vi "Acquisition Example.vi"() -> ()   [LabVIEW 2025, in "GettingStarted_Acq_148X_Host.lvlib"]
uses:
  GettingStarted_Acq_148X_Host.lvlib
  Common/Types/Packet Table.ctl
  <instrlib>/FlexRIO/CSI-2/v2/Common/Types/LLP Data Type.ctl
  <vilib>/userDefined/Silver/nirio_resource_slv.ctl
  Types/CSI-2 Data Source.ctl
  Common/Types/Serial Channel Configuration.ctl
  <instrlib>/FlexRIO/CSI-2/v2/FPGA/Types/Display Parameters.ctl
  Common/Types/RAW Interpretation for Display.ctl
  <instrlib>/FlexRIO/CSI-2/v2/FPGA/Types/Timestamp ID.ctl
  Common/Types/GPIO Filter.ctl
  FPGA/Common/Types/SerDes Identifier.ctl
  <instrlib>/FlexRIO/CSI-2/v2/FPGA/Types/GPIO Bank.ctl
  <vilib>/vision/Image Controls.llb/IMAQ Image.ctl
  <vilib>/Utility/miscctls.llb/LVRowAndColumnUnsignedTypeDef.ctl
  <instrlib>/FlexRIO/API/Host/v1/NI FlexRIO/API/Wait for PoC Safe to Disconnect Channels Array.vi
  <vilib>/FPGAPlugInAG/Dynamic/niLvFpga_Close_Dynamic.vi
  <vilib>/rvi/interface/nirviCloseFPGA/nirviCloseFPGA.xnode
  <instrlib>/FlexRIO/API/Host/v1/NI FlexRIO API v1.lvlib
  Common/GettingStarted_Common_148X_Host.lvlib
  <instrlib>/FlexRIO/CSI-2/v2/Common/NI CSI-2 API Common v2.lvlib
  <instrlib>/FlexRIO/CSI-2/v2/FPGA/NI CSI-2 API FPGA v2.lvlib
  FPGA/Common/GettingStarted_Common_148X_FPGA.lvlib
panel:
  in  "Array":u8[](array[numeric])
  out "Acquisition Stopped":bool
  in  "Configuration":T1(tab)
  in  "Logged Packets to Display":i64=1400
  in  "Log Packets to Disk":bool
  in  "Bitfile Path":path=path "C:/dev/hardware-validation/src/labview/auto-vision/Automotive Vision/1487 HIHO GSE/FPGA Bitfiles/PXIe_1487_4_In_4_Out_Acq_Tap.lvbitx"
  in  "TDMS File Directory":path
  in  "RIO Device":T2="PXI1Slot2"
  in  "Display Acquired Images":bool=TRUE
  in  "Log I2C to Disk":bool
  in  "Log GPIO to Disk":bool
  in  "Channel Configurations":T3[](array[typedef])=[{"Serial Channel"="SI1", "FPGA Display Parameters"={"virtual channel"=0.0, "payload data type"=enum."RAW 8", "frame skip count"=0, "line skip count"=0, "pixel skip count"=0.0}, "RAW Display Parameters"={"Interpretation"=enum."Grayscale", "Bayer Parameters"={"Pattern"=3, "Algorithm"=0, "Red Gain"=1.0, "Green Gain"=1.0, "Blue Gain"=1.0}}}] {"RAW Display Parameters"."Bayer Parameters"."Blue Gain" min=0.0 max=3.99 step=0.1 format="%_4g"; "RAW Display Parameters"."Bayer Parameters"."Green Gain" min=0.0 max=3.99 step=0.1 format="%_4g"; "RAW Display Parameters"."Bayer Parameters"."Red Gain" min=0.0 max=3.99 step=0.1 format="%_4g"; "RAW Display Parameters"."Bayer Parameters"."Algorithm" items=["Bilinear", "VNG"]; "RAW Display Parameters"."Bayer Parameters"."Pattern" items=["GB", "GR", "BG", "RG"]}
  in  "CSI-2 Data Source":T7=1 items=["Raw", "Corrected"]
  in  "Configuration Script":path=path "C:/dev/hardware-validation/src/labview/auto-vision/Automotive Vision/1487 HIHO GSE/scripts/Image Receiver Scripts/9296A_RAW8.cpp"
  in  "Acquisition Duration (s)":dbl=1.0 format="%#_13g"
  in  "Continuous Acquisition":bool=TRUE
  in  "Data Type Filter":T5[](array[typedef])
  in  "Virtual Channel Filter":fxp<+,4,4>[](array[numeric])
  in  "Invert Data Type Filter":bool
  in  "Invert Virtual Channel Filter":bool
  in  "Enable First and Last Packet Select":bool=TRUE
  in  "Stop Timeout (s)":dbl=1.0
  in  "First Packet Data Type Select":T5
  in  "Last Packet Data Type Select":T5=enum."Frame End"
  in  "Serial Input Active Lane Count":i32(ring)=4 items=["1 Lane"=1, "2 Lanes"=2, "4 Lanes"=4]
  in  "Reference Clock Frequency (Hz)":dbl=25000000.0 format="%#_6p"
  in  "Power Over Coax Source":i32(ring) items=["None", "Internal", "Auxiliary"]
  in  "timestamp filter":T8[](array[typedef])
  in  "GPIO to Display":T9[](array[typedef])
  in  "GPIO Bank Select":T10
  in  "Write GPIO":bool
  in  "GPIO Bank Write":T11
  out "GPIO Bank Read":T11
  out "Acquisition Duration (s)":dbl format="%.1f"
  out "Acquisition In Progress":bool
  out "Power Over Coax Voltage (V)":dbl[](array[numeric]) format="%#.2pV"
  out "Power Over Coax Current (A)":dbl[](array[numeric]) format="%#.2pA"
  in  "Acquired Serial Input Channel Data":T12(tab)
  out "Source Rate (fps)(1st Display)":dbl
  out "Update Rate (fps)(1st Display)":dbl
  in  "Serial Channel (1st Display)":fxp<+,3,3>
  out "1st channel display":T13(plugin-control)
  out "Source Rate (fps)(2nd Display)":dbl
  out "Update Rate (fps)(2nd Display)":dbl
  out "2nd channel display":T13(plugin-control)
  in  "Serial Channel (2nd Display)":fxp<+,3,3>
  out "Bytes Acquired (1st Channel)":i64 format="%#.6p"
  out "Acquired Packets (1st Channel)":T14
  out "Packets Logged (1st Channel)":i64
  out "Bytes Acquired (2nd Channel)":i64 format="%#.6p"
  out "Acquired Packets (2nd Channel)":T14
  out "Packets Logged (2nd Channel)":i64
  out "I2C Timestamps":T14
  out "GPIO Timestamps Waveform":digitalwaveform[](graph)
  out "Error Parsing GPIO Timestamps":bool
  out "Power Over Coax Source In Range":bool[](array[boolean])
  in  "Stop Acquisition":bool
  out "Error Out":errorcluster
  # "Overview: Configure an acquisition for a CSI-2 sensor and transfer the acquired data and timestamps to disk.  \nInstructions: Visit https://ni.com/r/automotive-camera-module-ref for tutorials and reference material on using this example with the PXIe-148X."
  # "Configuration Settings"
  # "Data Output"
  # "Resource Configuration"
  # "Data Output Configuration"
  # "Channel Configuration"
  # "Acquisition Configuration"
  # "First and Last Packet Select Configuration"
  # "Packet Filter Configuration"
  # "Power Over Coax Configuration"
  # "Clocking Configuration"
  # "I2C Timestamp Configuration"
  # "The timestamp filters listed correspond to the I2C traffic for a specific serial channel:\n\nUser24 = SI0\nUser25 = SI1\nUser26 = SI2\nUser27 = SI3\nUser28 = SI4\nUser29 = SI5\nUser30 = SI6\nUser31 = SI7"
  # "GPIO Configuration"
  # "* For additional packet viewing capability, use GettingStarted_Common_148X_Host.lvlib->TDMS File Viewer.vi"
  # "* For additional packet viewing capability, use GettingStarted_Common_148X_Host.lvlib->TDMS File Viewer.vi"
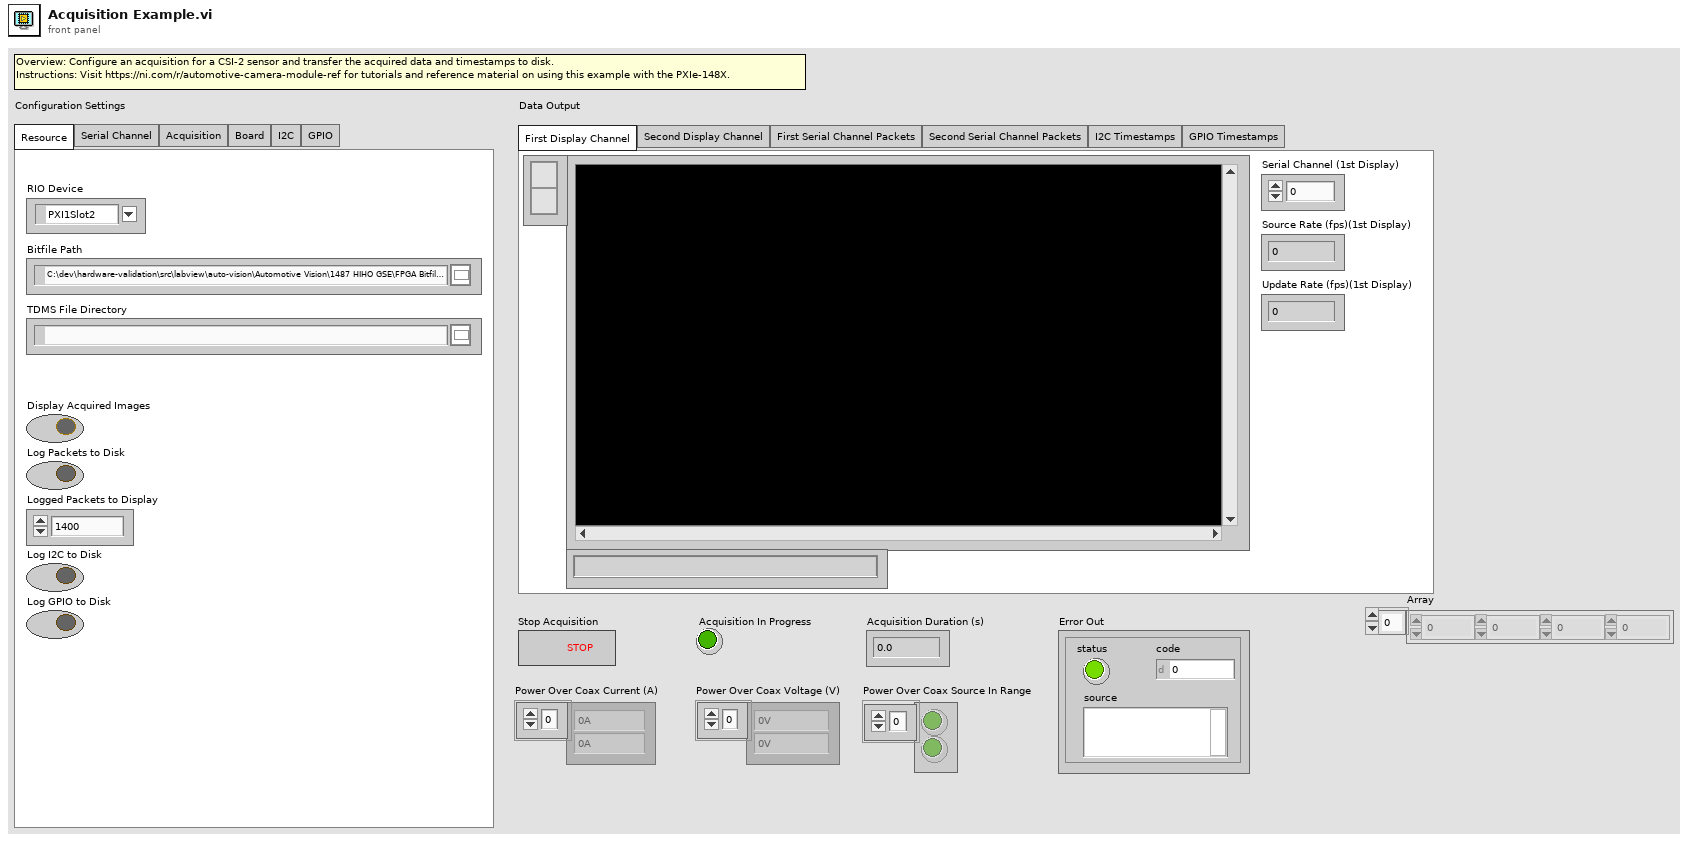
[diagram p1: front panel]
types:
  T1 = enum32{"Resource", "Serial Channel", "Acquisition", "Board", "I2C", "GPIO"}
  T2 = typedef "nirio_resource_slv.ctl" = tag
  T3 = typedef "GettingStarted_Common_148X_Host.lvlib/Serial Channel Configuration.ctl" = cluster{"Serial Channel":string, "FPGA Display Parameters":T4, "RAW Display Parameters":cluster{"Interpretation":T6, "Bayer Parameters":cluster{"Pattern":i32, "Algorithm":i32, "Red Gain":dbl, "Green Gain":dbl, "Blue Gain":dbl}}}
  T4 = typedef "NI CSI-2 API FPGA v2.lvlib/Display Parameters.ctl" = cluster{"virtual channel":fxp<+,4,4>, "payload data type":T5, "frame skip count":u16, "line skip count":u8, "pixel skip count":fxp<+,5,5>}
  T5 = typedef "NI CSI-2 API Common v2.lvlib/LLP Data Type.ctl" = enum8{"Frame Start", "Frame End", "Line Start", "Line End", "End of Transmission", "Reserved 0", "Reserved 1", "Reserved 2", "Generic Short Packet 1", "Generic Short Packet 2", "Generic Short Packet 3", "Generic Short Packet 4", "Generic Short Packet 5", "Generic Short Packet 6", "Generic Short Packet 7", "Generic Short Packet 8", "Null", "Blanking Data", "Embedded 8-bit non Image Data", "Generic Long Packet 1", "Generic Long Packet 2", "Generic Long Packet 3", "Generic Long Packet 4", "Reserved 3", "YUV420 8-bit", "YUV420 10-bit", "Legacy YUV420 8-bit", "Reserved 4", "YUV420 8-bit Chroma Shifted", "YUV420 10-bit Chroma Shifted", "YUV422 8-bit", "YUV422 10-bit", "RGB444", "RGB555", "RGB565", "RGB666", "RGB888", "Reserved 5", "Reserved 6", "RAW 24", "RAW 6", "RAW 7", "RAW 8", "RAW 10", "RAW 12", "RAW 14", "RAW 16", "RAW 20", "User Defined 8-bit Data 1", "User Defined 8-bit Data 2", "User Defined 8-bit Data 3", "User Defined 8-bit Data 4", "User Defined 8-bit Data 5", "User Defined 8-bit Data 6", "User Defined 8-bit Data 7", "User Defined 8-bit Data 8", "USL Command", "Reserved 7", "Reserved 8", "Reserved 9", "Reserved 10", "Reserved 11", "Reserved 12", "LRTE EPD Spacer"}
  T6 = typedef "GettingStarted_Common_148X_Host.lvlib/RAW Interpretation for Display.ctl" = enum16{"Grayscale", "Bayer", "RGB", "YUV422", "YUV420", "Legacy YUV420"}
  T7 = typedef "GettingStarted_Acq_148X_Host.lvlib/CSI-2 Data Source.ctl" = u16
  T8 = typedef "NI CSI-2 API FPGA v2.lvlib/Timestamp ID.ctl" = enum8{"SI0 LLP", "SI1 LLP", "SI2 LLP", "SI3 LLP", "SI4 LLP", "SI5 LLP", "SI6 LLP", "SI7 LLP", "SO0 LLP", "SO1 LLP", "SO2 LLP", "SO3 LLP", "SO4 LLP", "SO5 LLP", "SO6 LLP", "SO7 LLP", "Ser0 GPIO Bank", "Ser1 GPIO Bank", "Ser2 GPIO Bank", "Ser3 GPIO Bank", "Ser4 GPIO Bank", "Ser5 GPIO Bank", "Ser6 GPIO Bank", "Ser7 GPIO Bank", "Des0 GPIO Bank", "Des1 GPIO Bank", "Des2 GPIO Bank", "Des3 GPIO Bank", "Des4 GPIO Bank", "Des5 GPIO Bank", "Des6 GPIO Bank", "Des7 GPIO Bank", "User0", "User1", "User2", "User3", "User4", "User5", "User6", "User7", "User8", "User9", "User10", "User11", "User12", "User13", "User14", "User15", "User16", "User17", "User18", "User19", "User20", "User21", "User22", "User23", "User24", "User25", "User26", "User27", "User28", "User29", "User30", "User31"}
  T9 = typedef "GettingStarted_Common_148X_Host.lvlib/GPIO Filter.ctl" = cluster{"GPIO Bank":T8, "GPIO Number":i32}
  T10 = typedef "GettingStarted_Common_148X_FPGA.lvlib/SerDes Identifier.ctl" = enum8{"None", "SI 0 Deserializer", "SI 1 Deserializer", "SI 2 Deserializer", "SI 3 Deserializer", "SI 4 Deserializer", "SI 5 Deserializer", "SI 6 Deserializer", "SI 7 Deserializer", "SO 0 Serializer", "SO 1 Serializer", "SO 2 Serializer", "SO 3 Serializer", "SO 4 Serializer", "SO 5 Serializer", "SO 6 Serializer", "SO 7 Serializer", "SI 0 SI 1 Deserializer", "SI 2 SI 3 Deserializer", "SI 4 SI 5 Deserializer", "SI 6 SI 7 Deserializer"}
  T11 = typedef "NI CSI-2 API FPGA v2.lvlib/GPIO Bank.ctl" = cluster{"GPIO 0":bool, "GPIO 1":bool, "GPIO 2":bool, "GPIO 3":bool, "GPIO 4":bool, "GPIO 5":bool, "GPIO 6":bool, "GPIO 7":bool, "GPIO 8":bool, "GPIO 9":bool, "GPIO 10":bool}
  T12 = enum32{"First Display Channel", "Second Display Channel", "First Serial Channel Packets", "Second Serial Channel Packets", "I2C Timestamps", "GPIO Timestamps"}
  T13 = typedef "IMAQ Image.ctl" = refnum<image>
  T14 = typedef "GettingStarted_Common_148X_Host.lvlib/Packet Table.ctl" = string[][]
  T15 = typedef "LVRowAndColumnUnsignedTypeDef.ctl" = cluster{"Row":u32, "Column":u32}
  T16 = typedef "GettingStarted_Common_148X_Host.lvlib/Serial Channel Display Parameters.ctl" = cluster{"images":cluster{"grayscale":T13, "color":T13}, "RAW parameters":cluster{"interpretation":T6, "bayer parameters":cluster{"pattern":i32, "algorithm":i32, "red gain":dbl, "green gain":dbl, "blue gain":dbl}}}
  T17 = cluster{"Source Rate (fps)(1st Display)":refnum<vi>, "Update Rate (fps)(1st Display)":refnum<vi>}
  T18 = cluster{"Source Rate (fps)(2nd Display)":refnum<vi>, "Update Rate (fps)(2nd Display)":refnum<vi>}
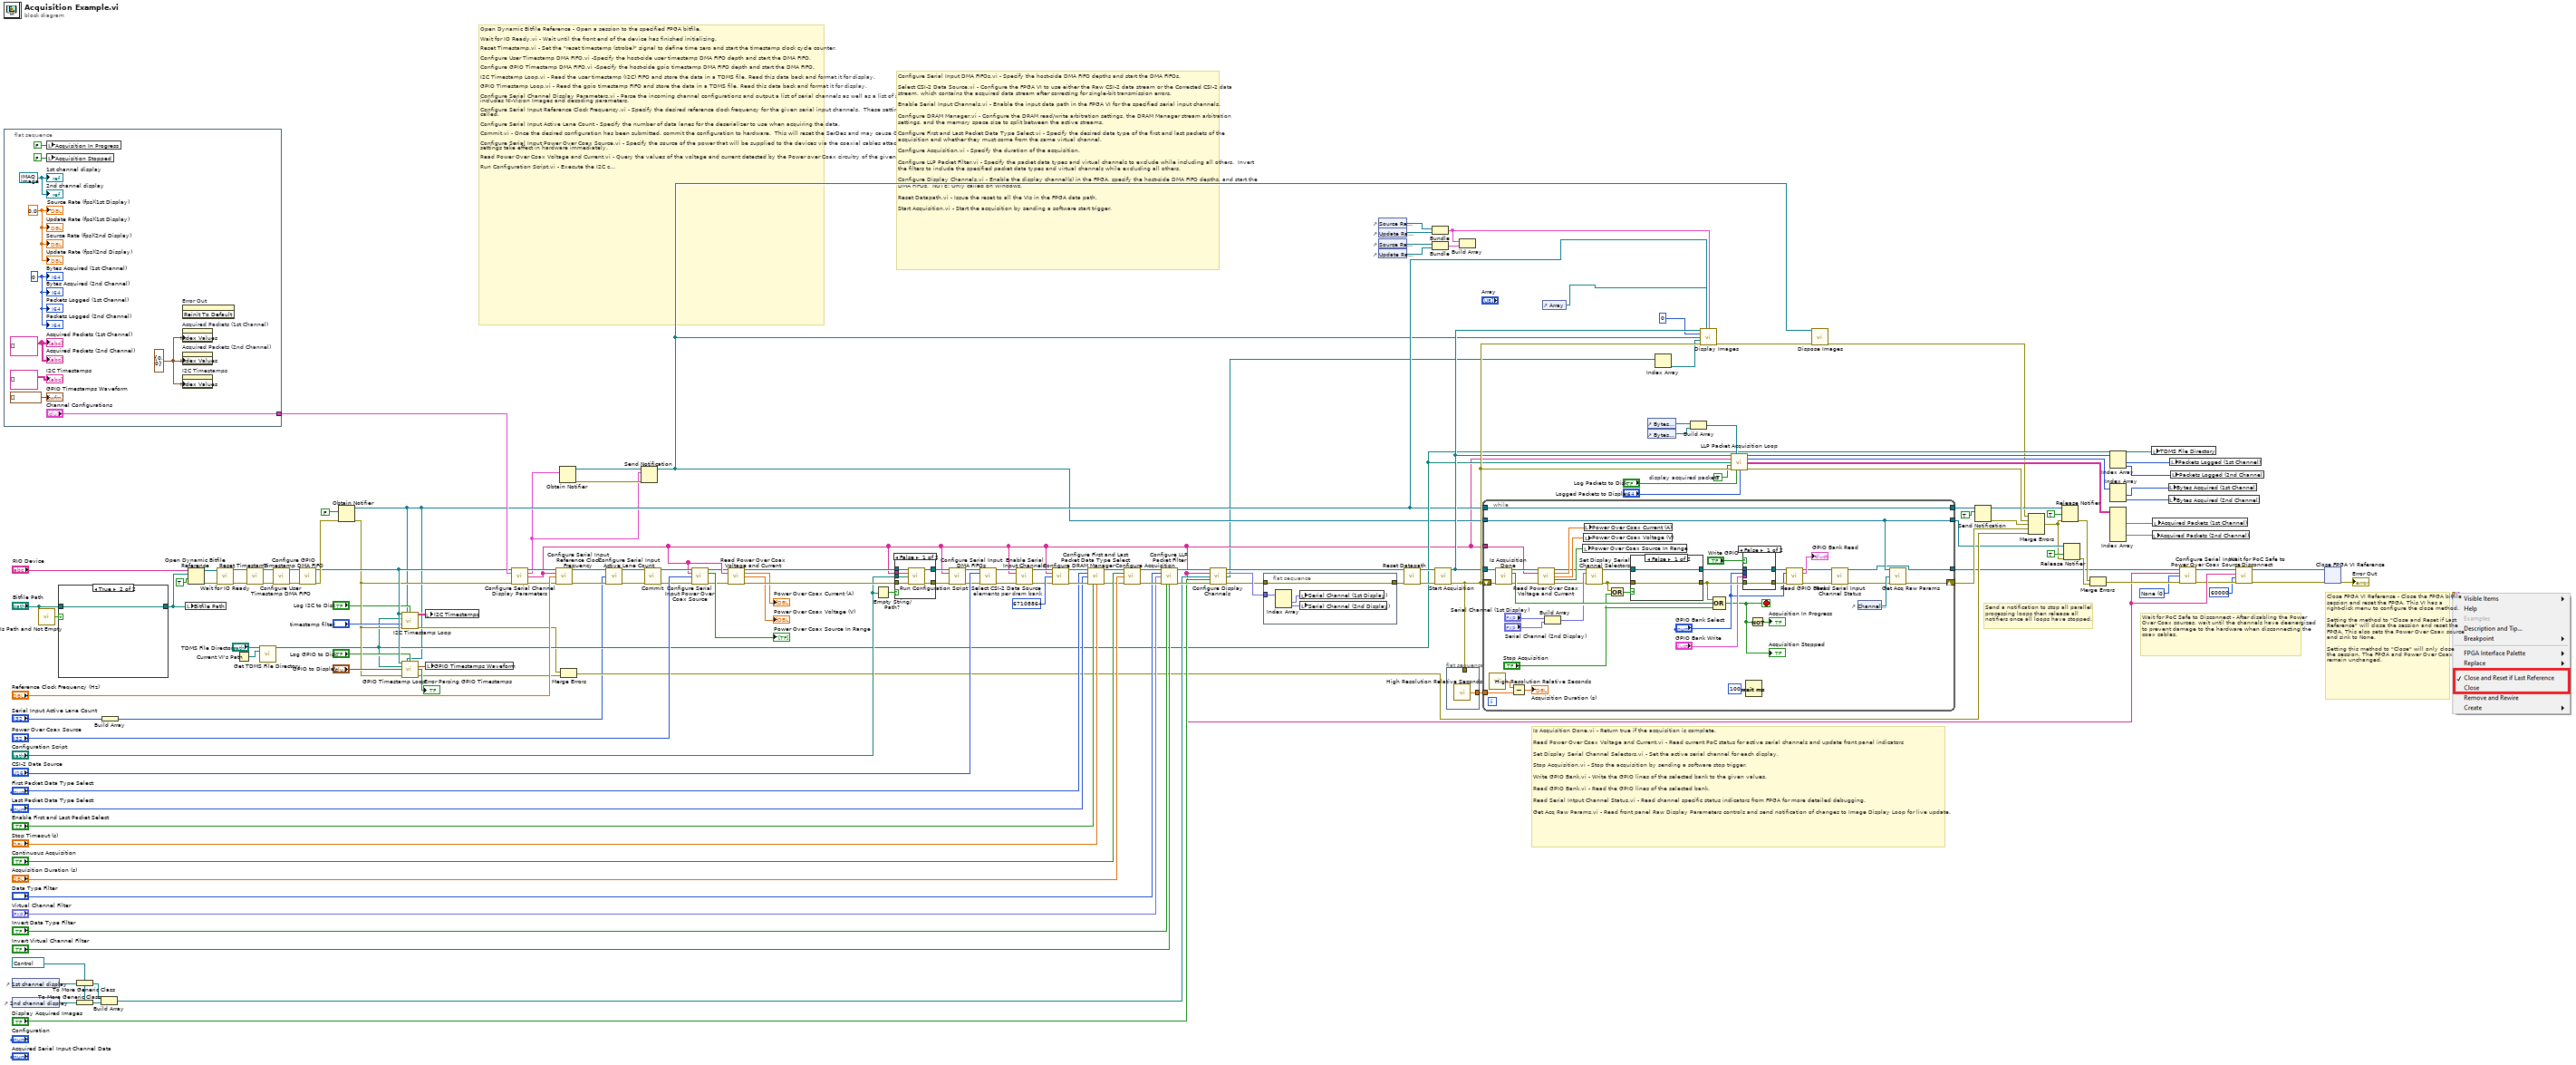
[diagram p0: block diagram]
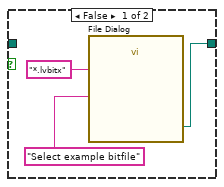
[diagram p2: hidden frame]
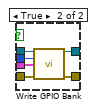
[diagram p4: hidden frame]
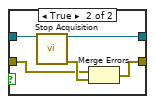
[diagram p5: hidden frame]
diagram:
  w9 = 0 items=["None", "Internal", "Auxiliary"] ("power over coax source")
  w36 = TRUE  # display acquired packets
  w85 = refnum<vi> refnum ("image display reference")
  w150 = u32 67108864  # elements per dram bank
  # "Wait for PoC Safe to Disconnect - After disabling the Power Over Coax sources, wait until the channels have deenergized to prevent damage to the hardware when disconnecting the coax cables."
  # "Send a notification to stop all parallel processing loops then release all notifiers once all loops have stopped."
  # "Configure Serial Input DMA FIFOs.vi - Specify the host-side DMA FIFO depths and start the DMA FIFOs.\n\nSelect CSI-2 Data Source.vi - Configure the FPGA VI to use either the Raw CSI-2 data stream or the Corrected CSI-2 data stream, which contains the acquired data stream after correcting for single-bit transmission errors.\n\nEnable Serial Input Channels.vi - Enable the input data path in the FPGA VI for the specified serial input channels.\n\nConfigure DRAM Manager.vi - Configure the DRAM read/write arbitration settings, the DRAM Manager stream arbitration settings, and the memory space size to split between the active streams.\n\nConfigure First and Last Packet Data Type Select.vi - Specify the desired data type of the first and last packets of the acquisition and whether they must come from the same virtual channel.\n\nConfigure Acquisition.vi - Specify the duration of the acquisition.\n\nConfigure LLP Packet Filter.vi - Specify the packet data types and virtual channels to exclude while including all others.  Invert the filters to include the specified packet data types and virtual channels while excluding all others.\n\nConfigure Display Channels.vi - Enable the display channel(s) in the FPGA, specify the host-side DMA FIFO depths, and start the DMA FIFOs.  NOTE: Only called on Windows. \n\nReset Datapath.vi - Issue the reset to all the VIs in the FPGA data path.\n\nStart Acquisition.vi - Start the acquisition by sending a software start trigger."
  # "Close FPGA VI Reference - Close the FPGA bitfile session and reset the FPGA. This VI has a right-click menu to configure the close method. \n\nSetting the method to \"Close and Reset if Last Reference\" will close the session and reset the FPGA. This also sets the Power Over Coax source and sink to None.\n\nSetting this method to \"Close\" will only close the session. The FPGA and Power Over Coax remain unchanged."
  # "Open Dynamic Bitfile Reference - Open a session to the specified FPGA bitfile.\n\nWait for IO Ready.vi - Wait until the front end of the device has finished initializing.\n\nReset Timestamp.vi - Set the \"reset timestamp (strobe)\" signal to define time zero and start the timestamp clock cycle counter.\n\nConfigure User Timestamp DMA FIFO.vi -Specify the host-side user timestamp DMA FIFO depth and start the DMA FIFO.\n\nConfigure GPIO Timestamp DMA FIFO.vi -Specify the host-side gpio timestamp DMA FIFO depth and start the DMA FIFO.\n\nI2C Timestamp Loop.vi - Read the user timestamp (I2C) FIFO and store the data in a TDMS file. Read this data back and format it for display.\n\nGPIO Timestamp Loop.vi - Read the gpio timestamp FIFO and store the data in a TDMS file. Read this data back and format it for display.\n\nConfigure Serial Channel Display Parameters.vi - Parse the incoming channel configurations and output a list of serial channels as well as a list of serial channel display parameters, which includes NI-Vision Images and decoding parameters.\n\nConfigure Serial Input Reference Clock Frequency.vi - Specify the desired reference clock frequency for the given serial input channels.  These settings do not take effect until Commit.vi is called.\n\nConfigure Serial Input Active Lane Count - Specify the number of data lanes for the deserializer to use when acquiring the data. \n\nCommit.vi - Once the desired configuration has been submitted, commit the configuration to hardware.  This will reset the SerDes and may cause GPIO lines to toggle. \n\nConfigure Serial Input Power Over Coax Source.vi - Specify the source of the power that will be supplied to the devices via the coaxial cables attached to the given serial input channels.  These settings take effect in hardware immediately.\n\nRead Power Over Coax Voltage and Current.vi - Query the values of the voltage and current detected by the Power over Coax circuitry of the given serial channels.\n\nRun Configuration Script.vi - Execute the I2C commands in the specified script file for the given serial channels.  The script is used to configure the serializer, deserializer, or other I2C slave device, such as the image sensor."
  # "Is Acquisition Done.vi - Return true if the acquisition is complete.\n\nRead Power Over Coax Voltage and Current.vi - Read current PoC status for active serial channels and update front panel indicators \n\nSet Display Serial Channel Selectors.vi - Set the active serial channel for each display.\n\nStop Acquisition.vi - Stop the acquisition by sending a software stop trigger.\n\nWrite GPIO Bank.vi - Write the GPIO lines of the selected bank to the given values.\n\nRead GPIO Bank.vi - Read the GPIO lines of the selected bank.\n\nRead Serial Intput Channel Status.vi - Read channel specific status indicators from FPGA for more detailed debugging.\n\nGet Acq Raw Params.vi - Read front panel Raw Display Parameters controls and send notification of changes to Image Display Loop for live update."
  n1 = flat-sequence {
    tunnel: ["Channel Configurations"] -> w98
    frame #0 {
      w151 = T15 {"Row"=0, "Column"=0} ("Index Values")
      w158 = T14 [] ("Acquired Packets (1st Channel)")
      w154 = 0 ("Number of Packets Acquired (1st Channel)")
      w157 = 0.0 ("display fps (2nd display)")
      w160 = T13 refnum ("first channel display")
      n2 = local write "Acquisition In Progress"(FALSE ("Acquisition In Progress")) -> ()
      n3 = local write "Acquisition Stopped"(FALSE ("Acquisition Stopped")) -> ()
      n4 = invoke on="Error Out" class="Clust (strict)" method="Reinit To Default"() -> ()  [unwired: 3 in, 3 out]
      n5 = property on="Acquired Packets (1st Channel)" class="Tbl (strict)"("Index Values"=w151) -> ()  [unwired: 2 in, 2 out]
      n6 = property on="Acquired Packets (2nd Channel)" class="Tbl (strict)"("Index Values"=w151) -> ()  [unwired: 2 in, 2 out]
      n7 = property on="I2C Timestamps" class="Tbl (strict)"("Index Values"=w151) -> ()  [unwired: 2 in, 2 out]
      "1st channel display" <- w160
      "2nd channel display" <- w160
      "Update Rate (fps)(1st Display)" <- w157
      "Update Rate (fps)(2nd Display)" <- w157
      "Acquired Packets (1st Channel)" <- w158
      "Packets Logged (1st Channel)" <- w154
      "Acquired Packets (2nd Channel)" <- w158
      "Packets Logged (2nd Channel)" <- w154
      "Source Rate (fps)(1st Display)" <- w157
      "Source Rate (fps)(2nd Display)" <- w157
      "GPIO Timestamps Waveform" <- digitalwaveform[] [] ("GPIO Timestamps Waveform")
      "I2C Timestamps" <- T14 [] ("I2C Timestamps 2")
      "Bytes Acquired (1st Channel)" <- w154
      "Bytes Acquired (2nd Channel)" <- w154
    }
  }
  n8 = control-ref of="1st channel display"() -> (w95:refnum<vi>)
  n9 = control-ref of="2nd channel display"() -> (w93:refnum<vi>)
  n10 = call <vilib>:"Is Path and Not Empty.vi"("path"="Bitfile Path") -> ("Is Path and Not Empty?"=w132:bool)  [unwired: 4 in]
  n11 = case shown="True" w132 {
    tunnel: "Bitfile Path" -> [_ w164]
    tunnel: [w162 w164] -> w131
    frame False {
      n12 = call "File Dialog"("prompt"="Select example bitfile", "pattern (all files)"="*.lvbitx") -> ("selected path"=w162:path)  [unwired: 10 in, 3 out]
    }
    frame True {
    }
  }
  n13 = To More Generic Class(target class=w85, reference=w95) -> (generic class reference=w94:refnum<vi>)
  n14 = To More Generic Class(target class=w85, reference=w93) -> (generic class reference=w92:refnum<vi>)
  n15 = Build Array(w94, w92) -> (w90:refnum<vi>[])
  n16 = Build Array("Serial Input Active Lane Count") -> (w27:i32[])
  n17 = local write "Bitfile Path"(w131) -> ()
  n18 = Open Dynamic Bitfile Reference(0:"RIO Device", 1:w131, 2:TRUE ("Run When Loaded")) -> (5:w129:refnum<k20>, 8:w130:errorcluster)  [unwired: 2 in]
  n19 = call <instrlib>:"Wait for IO Ready.vi"("fpga interface in"=w129, "error in"=w130) -> ("fpga interface out"=w65:refnum<k20>, "error out"=w66:errorcluster)  [unwired: 10 in, 2 out]
  n20 = Current VI's Path() -> (path=w102:path)
  n21 = call "Reset Timestamp.vi"("fpga interface in"=w65, "error in (no error)"=w66) -> ("fpga interface out"=w55:refnum<k20>, "error out"=w54:errorcluster)  [unwired: 12 in]
  n22 = call "Get TDMS File Directory.vi"("tdms file directory in"="TDMS File Directory", "calling vi path"=w102) -> ("tdms file directory out"=w40:path)  [unwired: 13 in]
  n23 = call "Configure User Timestamp DMA FIFO.vi"("fpga interface in"=w55, "error in (no error)"=w54) -> ("fpga interface out"=w53:refnum<k20>, "error out"=w52:errorcluster)  [unwired: 12 in]
  n24 = call "Configure GPIO Timestamp DMA FIFO.vi"("fpga interface in"=w53, "error in (no error)"=w52) -> ("fpga interface out"=w49:refnum<k20>, "error out"=w51:errorcluster)  [unwired: 12 in]
  n25 = Obtain Notifier(notification data type=FALSE ("result"), error in (no error)=w51) -> (notifier out=w26:refnum<notifier>, error out=w43:errorcluster)  [unwired: 2 in, 1 out]
  n26 = call "I2C Timestamp Loop.vi"("fpga interface in"=w49, "'stop' notifier"=w26, "log i2c to disk"="Log I2C to Disk", "tdms file directory"=w40, "timestamp filter"="timestamp filter", "error in (no error)"=w43) -> ("i2c data"=w48:string[][], "error out"=w38:errorcluster)  [unwired: 8 in]
  n27 = call "GPIO Timestamp Loop.vi"("fpga interface in"=w49, "'stop' notifier"=w26, "log gpio to disk"="Log GPIO to Disk", "tdms file directory"=w40, "gpio to display"="GPIO to Display", "error in (no error)"=w43) -> ("gpio timestamps waveform"=w47:digitalwaveform[], "error parsing gpio timestamps"=→"Error Parsing GPIO Timestamps":bool, "error out"=w37:errorcluster)  [unwired: 7 in]
  n28 = local write "I2C Timestamps"(w48) -> ()
  n29 = local write "GPIO Timestamps Waveform"(w47) -> ()
  n30 = call "Configure Serial Channel Display Parameters.vi"("fpga interface in"=w49, "serial channel configurations"=w98, "error in (no error)"=w43) -> ("fpga interface out"=w97:refnum<k20>, "serial channel display parameters"=w23:T16[], "serial channels"=w12:string[], "error out"=w96:errorcluster)  [unwired: 9 in]
  n31 = call "Configure Serial Input Reference Clock Frequency.vi"("fpga interface in"=w97, "serial input channels"=w12, "serial input reference clock frequency (Hz)"="Reference Clock Frequency (Hz)", "error in (no error)"=w96) -> ("fpga interface out"=w32:refnum<k20>, "error out"=w31:errorcluster)  [unwired: 10 in]
  n32 = Obtain Notifier(notification data type=w23) -> (notifier out=w25:refnum<notifier>, error out=w24:errorcluster)  [unwired: 3 in, 1 out]
  n33 = Merge Errors(w38, w37) -> (w33:errorcluster)
  n34 = call "Configure Serial Input Active Lane Count.vi"("fpga interface in"=w32, "serial input active lane counts"=w27, "error in (no error)"=w31) -> ("fpga interface out"=w30:refnum<k20>, "error out"=w29:errorcluster)  [unwired: 11 in]
  n35 = Send Notification(notification=w23, notifier=w25, error in (no error)=w24) -> (notifier out=w22:refnum<notifier>)  [unwired: 1 out]
  n36 = call <instrlib>:"Commit.vi"("fpga interface in"=w30, "error in"=w29) -> ("fpga interface out"=w136:refnum<k20>, "error out"=w137:errorcluster)  [unwired: 12 in]
  n37 = call "Configure Serial Input Power Over Coax Source.vi"("fpga interface in"=w136, "serial input channels"=w12, "power over coax source"="Power Over Coax Source", "error in (no error)"=w137) -> ("fpga interface out"=w10:refnum<k20>, "power over coax source in range"=→"Power Over Coax Source In Range":bool[], "error out"=w11:errorcluster)  [unwired: 9 in]
  n38 = call "Read Power Over Coax Voltage and Current.vi"("fpga interface in"=w10, "serial channels"=w12, "error in (no error)"=w11) -> ("fpga interface out"=w126:refnum<k20>, "current (A)"=→"Power Over Coax Current (A)":dbl[], "voltage (V)"=→"Power Over Coax Voltage (V)":dbl[], "error out"=w127:errorcluster)  [unwired: 8 in, 1 out]
  n39 = Empty String/Path?(string/path="Configuration Script") -> (empty?=w68:bool)
  n40 = case shown="False" w68 {
    tunnel: [w170 w171] -> w148
    tunnel: [w169 w172] -> w140
    tunnel: w127 -> [w168 w171]
    tunnel: w126 -> [w167 w172]
    tunnel: w12 -> [w166 _]
    tunnel: "Configuration Script" -> [w165 _]
    frame False {
      n41 = call "Run Configuration Script.vi"("fpga interface in"=w167, "serial channels"=w166, "configuration script"=w165, "error in (no error)"=w168) -> ("fpga interface out"=w169:refnum<k20>, "error out"=w170:errorcluster)  [unwired: 10 in]
    }
    frame True {
    }
  }
  n42 = call "Configure Serial Input DMA FIFOs.vi"("fpga interface in"=w140, "serial channels"=w12, "error in (no error)"=w148) -> ("fpga interface out"=w118:refnum<k20>, "error out"=w115:errorcluster)  [unwired: 11 in]
  n43 = call "Select CSI-2 Data Source.vi"("fpga interface in"=w118, "csi-2 data source"="CSI-2 Data Source", "error in (no error)"=w115) -> ("fpga interface out"=w117:refnum<k20>, "error out"=w116:errorcluster)  [unwired: 11 in]
  n44 = call "Enable Serial Input Channels.vi"("fpga interface in"=w117, "serial input channels"=w12, "error in (no error)"=w116) -> ("fpga interface out"=w139:refnum<k20>, "error out"=w149:errorcluster)  [unwired: 11 in]
  n45 = call "Configure DRAM Manager.vi"("fpga interface in"=w139, "serial channels"=w12, "elements per dram bank"=w150, "error in (no error)"=w149) -> ("fpga interface out"=w111:refnum<k20>, "error out"=w114:errorcluster)  [unwired: 10 in]
  n46 = call "Configure First and Last Packet Data Type Select.vi"("fpga interface in"=w111, "first packet data type select"="First Packet Data Type Select", "last packet data type select"="Last Packet Data Type Select", "error in (no error)"=w114, "enable first and last packet select"="Enable First and Last Packet Select", "stop timeout (s)"="Stop Timeout (s)") -> ("fpga interface out"=w112:refnum<k20>, "error out"=w113:errorcluster)  [unwired: 8 in]
  n47 = call "Configure Acquisition.vi"("fpga interface in"=w112, "continuous acquisition (T)"="Continuous Acquisition", "acquisition duration (s)"="Acquisition Duration (s)", "error in (no error)"=w113) -> ("fpga interface out"=w145:refnum<k20>, "error out"=w146:errorcluster)  [unwired: 10 in]
  n48 = call "Configure LLP Packet Filter.vi"("fpga interface in"=w145, "data type filter"="Data Type Filter", "virtual channel filter"="Virtual Channel Filter", "error in (no error)"=w146, "invert data type filter"="Invert Data Type Filter", "invert virtual channel filter"="Invert Virtual Channel Filter") -> ("fpga interface out"=w99:refnum<k20>, "error out"=w91:errorcluster)  [unwired: 8 in]
  n49 = call "Configure Display Channels.vi"("fpga interface in"=w99, "serial channels"=w12, "display references in"=w90, "enable image display"="Display Acquired Images", "error in (no error)"=w91) -> ("fpga interface out"=w89:refnum<k20>, "display serial channels"=w88:fxp<+,3,3>[], "display references out"=w3:refnum<vi>[], "error out"=w87:errorcluster)  [unwired: 7 in]
  n50 = flat-sequence {
    tunnel: w88 -> [w174]
    tunnel: w87 -> [w173]
    tunnel: [w173] -> w86
    frame #0 {
      n51 = Index Array(array=w174) -> (element #1=w176:fxp<+,3,3>, element #2=w175:fxp<+,3,3>)  [unwired: 2 in]
      n52 = local write "Serial Channel (1st Display)"(w176) -> ()
      n53 = local write "Serial Channel (2nd Display)"(w175) -> ()
    }
  }
  n54 = control-ref of="Source Rate (fps)(1st Display)"() -> (w78:refnum<vi>)
  n55 = control-ref of="Update Rate (fps)(1st Display)"() -> (w79:refnum<vi>)
  n56 = control-ref of="Source Rate (fps)(2nd Display)"() -> (w77:refnum<vi>)
  n57 = control-ref of="Update Rate (fps)(2nd Display)"() -> (w76:refnum<vi>)
  n58 = call "Reset Datapath.vi"("fpga interface in"=w89, "error in (no error)"=w86) -> ("fpga interface out"=w147:refnum<k20>, "error out"=w50:errorcluster)  [unwired: 12 in]
  n59 = Bundle("Source Rate (fps)(1st Display)"=w78, "Update Rate (fps)(1st Display)"=w79) -> (w5:T17)  [unwired: 1 in]
  n60 = Bundle("Source Rate (fps)(2nd Display)"=w77, "Update Rate (fps)(2nd Display)"=w76) -> (w75:T18)  [unwired: 1 in]
  n61 = call "Start Acquisition.vi"("fpga interface in"=w147, "error in (no error)"=w50) -> ("fpga interface out"=w63:refnum<k20>, "error out"=w64:errorcluster)  [unwired: 12 in]
  n62 = flat-sequence {
    tunnel: [w177] -> w104
    tunnel: w64 -> [_]
    frame #0 {
      n63 = call <vilib>:"High Resolution Relative Seconds.vi"() -> ("relative seconds"=w177:dbl)
    }
  }
  n64 = Build Array(w5, w75) -> ()  [unwired: 1 out]
  n65 = while {
    shift-right: [w184] -> w34
    shift-left: w64 -> [w186]
    tunnel: w63 -> [w200]
    tunnel: w12 -> [w212]
    tunnel: w104 -> [w207]
    tunnel: w26 -> [w185]
    tunnel: [w185] -> w60
    tunnel: w22 -> [w182]
    tunnel: [w178] -> w16
    tunnel: [w182] -> w20
    stop <- w187 stop-if-true
    n66 = call <vilib>:"High Resolution Relative Seconds.vi"() -> ("relative seconds"=w208:dbl)
    n67 = call "Is Acquisition Done.vi"("fpga interface in"=w200, "error in (no error)"=w186) -> ("fpga interface out"=w213:refnum<k20>, "acquisition done"=w217:bool, "error out"=w214:errorcluster)  [unwired: 11 in]
    n68 = Subtract(x=w208, y=w207) -> (x-y=→"Acquisition Duration (s)":dbl)
    n69 = call "Read Power Over Coax Voltage and Current.vi"("fpga interface in"=w213, "serial channels"=w212, "error in (no error)"=w214) -> ("fpga interface out"=w202:refnum<k20>, "current (A)"=w211:dbl[], "voltage (V)"=w209:dbl[], "in range"=w210:bool[], "error out"=w201:errorcluster)  [unwired: 8 in]
    n70 = Build Array("Serial Channel (1st Display)", "Serial Channel (2nd Display)") -> (w203:fxp<+,3,3>[])
    n71 = local write "Power Over Coax Source In Range"(w210) -> ()
    n72 = local write "Power Over Coax Voltage (V)"(w209) -> ()
    n73 = local write "Power Over Coax Current (A)"(w211) -> ()
    n74 = call "Set Display Serial Channel Selectors.vi"("fpga interface in"=w202, "display serial channel selectors"=w203, "error in (no error)"=w201) -> ("fpga interface out"=w197:refnum<k20>, "error out"=w199:errorcluster)  [unwired: 11 in]
    n75 = Compound Arithmetic op=OR(w199, "Stop Acquisition") -> (w198:bool)
    n76 = case shown="False" w198 {
      tunnel: [w227 w229] -> w195
      tunnel: w199 -> [w227 w228]
      tunnel: [w226 w231] -> w196
      tunnel: w197 -> [w226 w230]
      frame False {
      }
      frame True {
        n77 = call "Stop Acquisition.vi"("fpga interface in"=w230) -> ("fpga interface out"=w231:refnum<k20>, "error out"=w232:errorcluster)  [unwired: 13 in]
        n78 = Merge Errors(w228, w232) -> (w229:errorcluster)
      }
    }
    n79 = Compound Arithmetic op=OR(w195, w217, "Stop Acquisition") -> (w187:bool)
    "Acquisition Stopped" <- w187
    n80 = case shown="False" "Write GPIO" {
      tunnel: w196 -> [w219 w225]
      tunnel: w195 -> [w218 w224]
      tunnel: "GPIO Bank Write" -> [_ w223]
      tunnel: [w219 w222] -> w193
      tunnel: [w218 w221] -> w192
      tunnel: "GPIO Bank Select" -> [_ w220]
      frame False {
      }
      frame True {
        n81 = call "Write GPIO Bank.vi"("fpga interface in"=w225, "gpio bank select"=w220, "gpio bank output"=w223, "error in (no error)"=w224) -> ("fpga interface out"=w222:refnum<k20>, "error out"=w221:errorcluster)  [unwired: 10 in]
      }
    }
    n82 = Wait (ms)(milliseconds to wait=u32 100) -> ()  [unwired: 1 out]
    n83 = Not(x=w187) -> (.not. x?=→"Acquisition In Progress":bool)
    n84 = call "Read GPIO Bank.vi"("fpga interface in"=w193, "gpio bank select"="GPIO Bank Select", "error in (no error)"=w192) -> ("fpga interface out"=w179:refnum<k20>, "gpio bank output"=→"GPIO Bank Read":T11, "error out"=w181:errorcluster)  [unwired: 10 in]
    n85 = call "Read Serial Input Channel Status.vi"("fpga interface in"=w179, "error in (no error)"=w181) -> ("fpga interface out"=w178:refnum<k20>, "error out"=w180:errorcluster)  [unwired: 11 in, 1 out]
    n86 = control-ref of="Channel Configurations"() -> (w183:refnum<vi>)
    n87 = call "Get Acq Raw Params.vi"("raw display notifier"=w182, "Channel Configurations"=w183, "error in (no error)"=w180) -> ("error out"=w184:errorcluster)  [unwired: 12 in]
  }
  n88 = control-ref of="Array"() -> (w1:refnum<vi>)
  n89 = control-ref of="Bytes Acquired (1st Channel)"() -> (w106:refnum<vi>)
  n90 = control-ref of="Bytes Acquired (2nd Channel)"() -> (w105:refnum<vi>)
  n91 = Index Array(array=w3) -> (element=w2:refnum<vi>)  [unwired: 1 in]
  n92 = Build Array(w106, w105) -> (w101:refnum<vi>[])
  n93 = call "Display Images.vi"("fpga interface in"=w63, "'stop' notifier"=w26, "rate references"=w5, "display channel number"=0, "raw display notifier"=w22, "display reference"=w2, "error in (no error)"=w64, "Ctl Refnum"=w1) -> ("error out"=w80:errorcluster)  [unwired: 6 in, 1 out]
  n94 = call "LLP Packet Acquisition Loop.vi"("fpga interface in"=w63, "bytes acquired references"=w101, "Serial Channels"=w12, "tdms file directory"=w40, "display acquired packets"=w36, "error in"=w64, "log to disk"="Log Packets to Disk", "num packets to read"="Logged Packets to Display") -> ("number of packets acquired"=w100:i64[], "number of bytes acquired"=w72:i64[], "display data"=w73:string[][][], "error out"=w61:errorcluster)  [unwired: 4 in]
  n95 = call "Dispose Images.vi"("raw display notifier"=w22, "error in (no error)"=w80) -> ("error out"=w39:errorcluster)  [unwired: 13 in]
  n96 = Send Notification(notification=TRUE, notifier=w60) -> (notifier out=w59:refnum<notifier>, error out=w58:errorcluster)  [unwired: 1 in]
  n97 = Merge Errors(w39, w61, w58, w34, w33) -> (w19:errorcluster)
  n98 = Release Notifier(notifier=w59, force destroy? (F)=TRUE, error in (no error)=w19) -> (error out=w18:errorcluster)  [unwired: 2 out]
  n99 = Release Notifier(notifier=w20, force destroy? (F)=TRUE, error in (no error)=w19) -> (error out=w17:errorcluster)  [unwired: 2 out]
  n100 = Merge Errors(w18, w17) -> (w15:errorcluster)
  n101 = Index Array(array=w100) -> (element #1=w84:i64, element #2=w83:i64)  [unwired: 2 in]
  n102 = Index Array(array=w72) -> (element #1=w71:i64, element #2=w70:i64)  [unwired: 2 in]
  n103 = Index Array(array=w73) -> (element #1=w82:string[][], element #2=w81:string[][])  [unwired: 6 in]
  n104 = local write "TDMS File Directory"(w40) -> ()
  n105 = local write "Acquired Packets (2nd Channel)"(w81) -> ()
  n106 = local write "Acquired Packets (1st Channel)"(w82) -> ()
  n107 = local write "Bytes Acquired (1st Channel)"(w71) -> ()
  n108 = local write "Bytes Acquired (2nd Channel)"(w70) -> ()
  n109 = local write "Packets Logged (1st Channel)"(w84) -> ()
  n110 = local write "Packets Logged (2nd Channel)"(w83) -> ()
  n111 = call "Configure Serial Input Power Over Coax Source.vi"("fpga interface in"=w16, "serial input channels"=w12, "power over coax source"=w9, "error in (no error)"=w15) -> ("fpga interface out"=w7:refnum<k20>, "error out"=w8:errorcluster)  [unwired: 9 in, 1 out]
  n112 = call-poly <instrlib>:"Wait for PoC Safe to Disconnect.vi"("error in"=w8, "Timeout (ms)"=60000 ("Wait for Safe to Disconnect Timeout (ms)"), "Channels"=w12, "fpga interface in"=w7) -> ("error out"=w14:errorcluster, "fpga interface out"=w13:refnum<k20>)  [unwired: 6 in]
  n113 = xnode ("Close FPGA VI Reference")("FPGA VI Reference In"=w13, "error in"=w14) -> ("error out"=→"Error Out":errorcluster)
